vi "testAndProjection.vi"() -> ()   [LabVIEW 2010]
panel:
  out "ZY view":u32[][](graph)
  out "XZ view":u32[][](graph)
  out "XY view":u32[][](graph)
  in  "scan specification":T1={"x amplitude"=100, "x resolution (pixels)"=28, "x offset fly-forward (iterations)"=50, "x offset fly-back (iterations)"=100, "y resolution (nr. of lines)"=80, "y step size"=30, "iterations per pixel"=5, "number of frames"=80, "y offset (pixels)"=0, "number of y-brake lines  (before y-fly-back)"=0, "number y-brake lines (after y-fly-back)"=40, "number of y-fly-back steps"=0, "lines per z step"=1, "number of z/intensity tuples"=228, "number of repetitions (volumes or planes)"=1000, "z step size derived"=32, "choose the beginning of z scan"=FALSE, "number of frames (settings)"=80, "FPGA trajectory?"=TRUE, "Pockels cell voltage (bits)"=0, "Vy min(bits)"=0, "Vz min(bits)"=0}
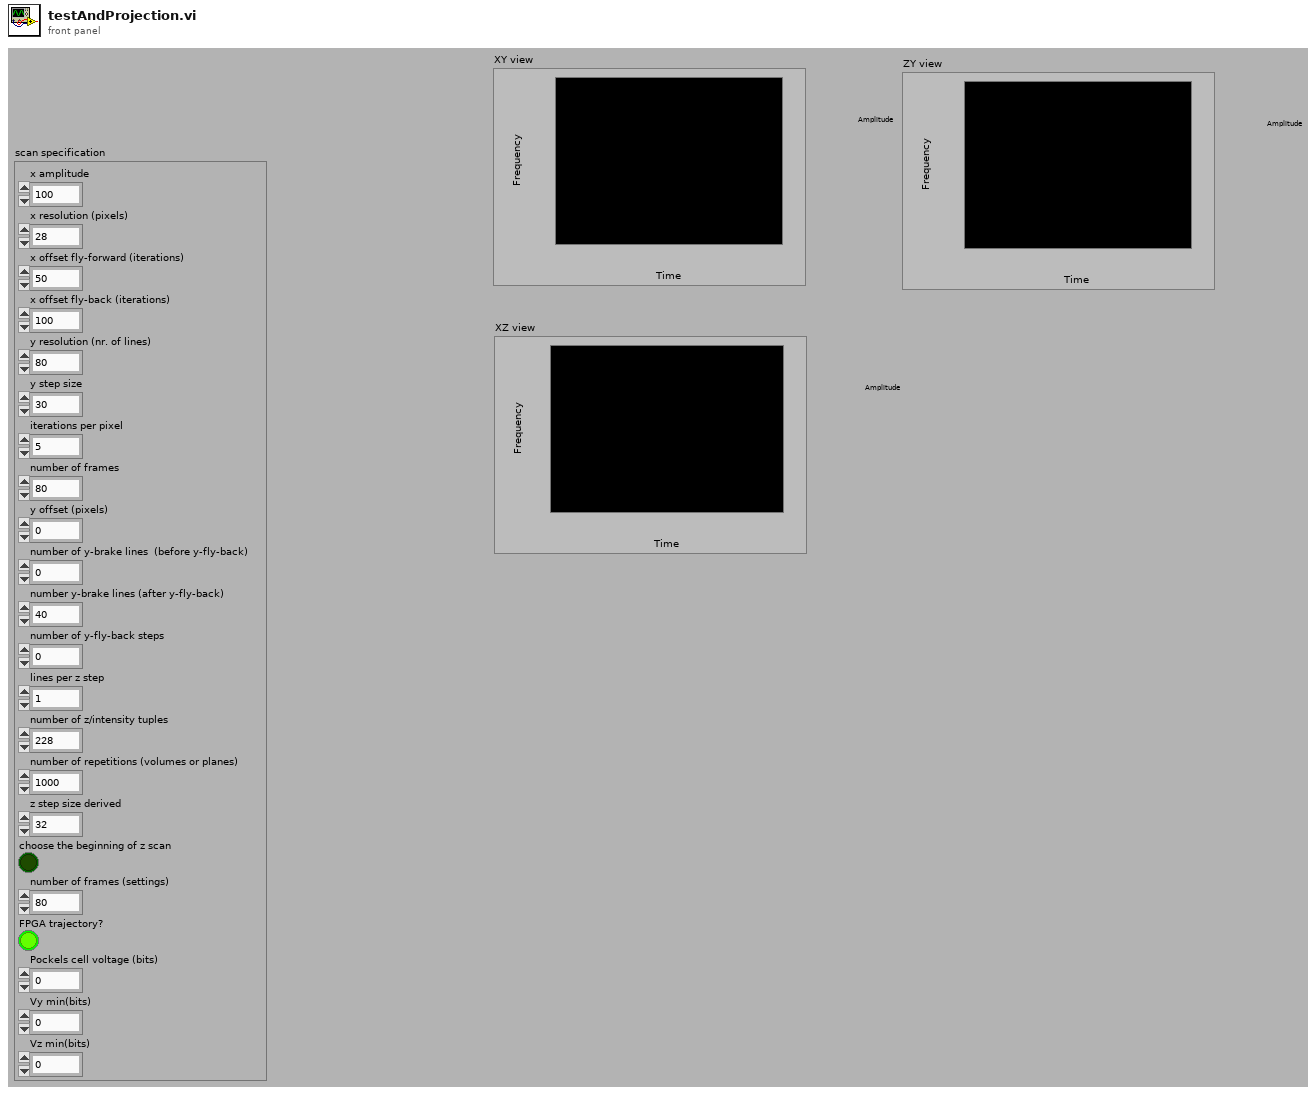
[diagram p1: front panel]
types:
  T1 = cluster{"x amplitude":u16, "x resolution (pixels)":u16, "x offset fly-forward (iterations)":u16, "x offset fly-back (iterations)":u16, "y resolution (nr. of lines)":u16, "y step size":u16, "iterations per pixel":u16, "number of frames":i32, "y offset (pixels)":u16, "number of y-brake lines  (before y-fly-back)":u16, "number y-brake lines (after y-fly-back)":u16, "number of y-fly-back steps":u16, "lines per z step":u16, "number of z/intensity tuples":u16, "number of repetitions (volumes or planes)":i32, "z step size derived":u16, "choose the beginning of z scan":bool, "number of frames (settings)":i32, "FPGA trajectory?":bool, "Pockels cell voltage (bits)":i16, "Vy min(bits)":i16, "Vz min(bits)":i16}
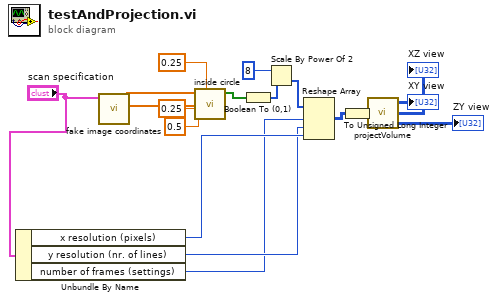
[diagram p0: block diagram]
diagram:
  n1 = Unbundle By Name("scan specification") -> ("x resolution (pixels)"=w4:u16, "y resolution (nr. of lines)"=w3:u16, "number of frames (settings)"=w2:i32)
  n2 = call "fake image coordinates.vi"("scan specification"="scan specification") -> ("ycoords"=w18:dbl[], "xcoords"=w8:dbl[])  [unwired: 8 in, 1 out]
  n3 = call "inside circle.vi"("r"=0.25, "yc"=0.5, "xc"=0.25, "ycoords"=w18, "xcoords"=w8) -> ("inside circle"=w14:bool[])  [unwired: 6 in]
  n4 = Boolean To (0,1)(Boolean=w14) -> (0, 1=w1:i16[])
  n5 = Scale By Power Of 2(n=8, x=w1) -> (x*2^n=w7:i16[])
  n6 = Reshape Array(w7, w2, w3, w4) -> (w12:i16[][][])
  n7 = To Unsigned Long Integer(number=w12) -> (unsigned 32bit integer=w5:u32[][][])
  n8 = call "projectVolume.vi"("input array"=w5) -> ("ZY view"=→"ZY view":u32[][], "XZ view"=→"XZ view":u32[][], "XY view"=→"XY view":u32[][])
